vi "onPlayVideo.vi"(8 "error in (no error)":errorcluster, 11 "CameraTestingUI in":refnum<class "CameraTestingUI.lvclass">) -> (0 "error out":errorcluster, 3 "CameraTestingUI out":refnum<class "CameraTestingUI.lvclass">)   [LabVIEW 2020, in "CameraTestingUI.lvlib" / "CameraTestingUI.lvclass"]
uses:
  CameraTestingUI.lvclass
  CameraTestingUI.lvclass/CameraTestingUI.ctl
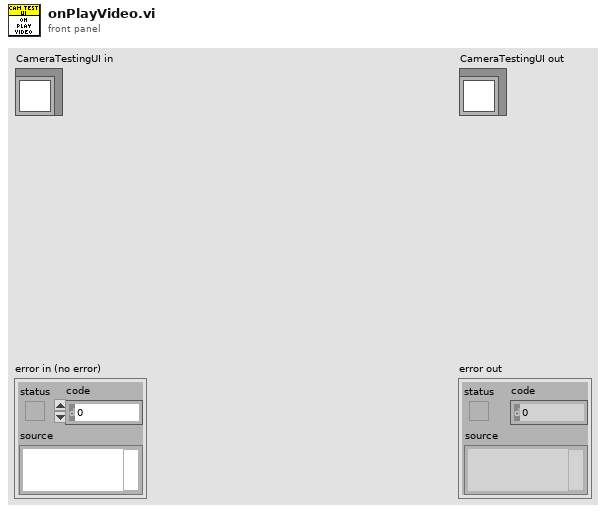
[diagram p1: front panel]
types:
  T1 = enum8{"Enabled", "Disabled", "Disabled and Grayed Out"}
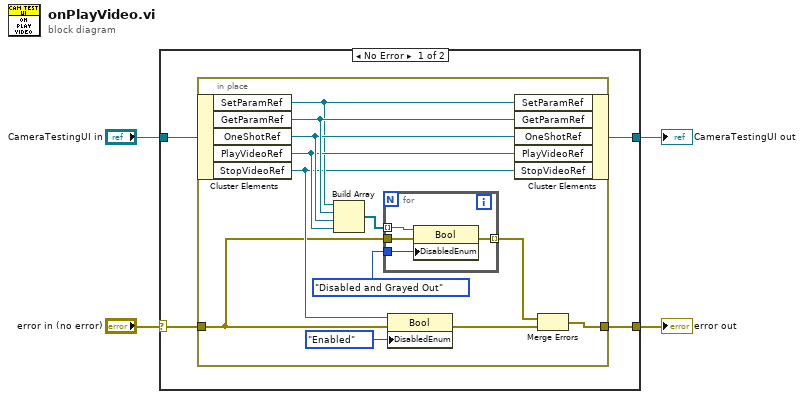
[diagram p0: block diagram]
diagram:
  n1 = case shown="No Error" "error in (no error)" {
    selector: "error in (no error)" -> [w6 w26]
    tunnel: [w5 w26] -> w3
    tunnel: [w7 w25] -> w1
    tunnel: "CameraTestingUI in" -> [w8 w25]
    frame No Error {
      n2 = in-place {
        in-place-border: w6 -> [w9]
        in-place-border: [w14] -> w5
        n3 = in-place-cluster #1(w8) -> ("SetParamRef"=w17:refnum<vi>, "GetParamRef"=w20:refnum<vi>, "OneShotRef"=w19:refnum<vi>, "PlayVideoRef"=w18:refnum<vi>, "StopVideoRef"=w13:refnum<vi>)
        n4 = Build Array(w17, w20, w19, w18) -> (w16:refnum<vi>[])
        n5 = for {
          tunnel: w16 -> [w24] mode=indexing
          tunnel: w9 -> [w23]
          tunnel: [w22] -> w15 mode=indexing
          tunnel: T1."Disabled and Grayed Out" ("Disabled") -> [w21]
          n6 = property class="Bool"(reference=w24, error in=w23, "DisabledEnum"=w21) -> (error out=w22:errorcluster)  [unwired: 1 out]
        }
        n7 = property class="Bool"(reference=w13, error in=w9, "DisabledEnum"=T1."Enabled" ("Disabled")) -> (error out=w10:errorcluster)  [unwired: 1 out]
        n8 = in-place-cluster #1("SetParamRef"=w17, "GetParamRef"=w20, "OneShotRef"=w19, "PlayVideoRef"=w18, "StopVideoRef"=w13) -> (w7:refnum<class "CameraTestingUI.lvclass">)
        n9 = Merge Errors(w15, w10) -> (w14:errorcluster)
      }
    }
    frame Error {
    }
  }
  "error out" <- w3
  "CameraTestingUI out" <- w1
